vi "TubeTemperatures.vi"(9 "Startup Temperature (ºC)":dbl, 10 "TubeTempEnum":T1, 11 "Current Thermistor Temperatures":dbl[](array[numeric])) -> (3 "Current Tube Temperatures":dbl[](array[numeric]))   [LabVIEW 2019]
doc: "TubeTempNow = (temp of therm-TubeTempBefore) * t/RC)\nWhere t = 1s and RC = 128s\n\nRC was calculated emperically by James Sprenke for CPVC tubing.\nThe reason that RC is used is because it closely models the response from the temperature\nconduction from the sounding tube. This is not a theoretical derivation but a close \napproximation."
uses:
  TubeTempEnum.ctl
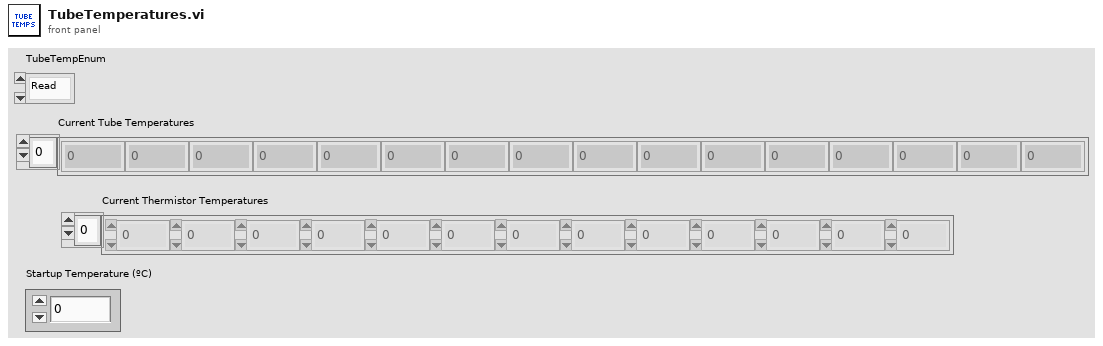
[diagram p1: front panel]
types:
  T1 = typedef "TubeTempEnum.ctl" = enum16{"Read", "Write", "Initialize"}
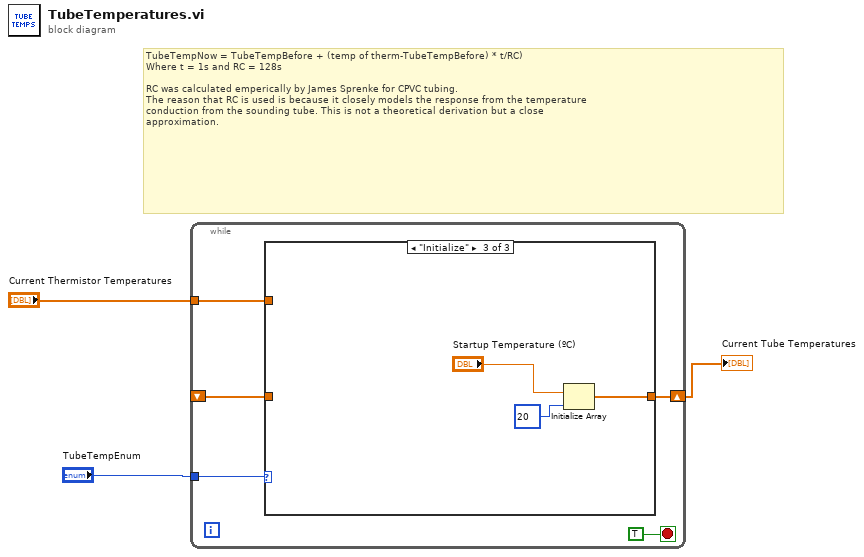
[diagram p0: block diagram]
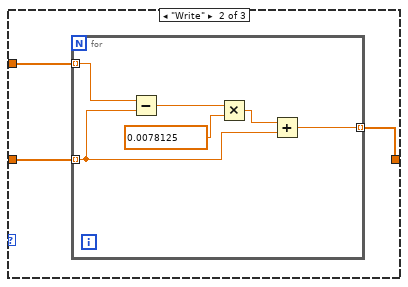
[diagram p3: hidden frame]
diagram:
  # "TubeTempNow = TubeTempBefore + (temp of therm-TubeTempBefore) * t/RC)\nWhere t = 1s and RC = 128s\n\nRC was calculated emperically by James Sprenke for CPVC tubing.\nThe reason that RC is used is because it closely models the response from the temperature\nconduction from the sounding tube. This is not a theoretical derivation but a close \napproximation."
  n1 = while {
    shift-right: [w5] -> w2
    shift-left: _ -> [w6]
    tunnel: "Current Thermistor Temperatures" -> [w7]
    tunnel: "TubeTempEnum" -> [w4]
    stop <- TRUE stop-if-true
    n2 = case shown="\"Initialize\"" w4 {
      tunnel: w7 -> [_ w12 _]
      tunnel: w6 -> [w9 w11 _]
      tunnel: [w9 w10 w19] -> w5
      frame "Read", Default {
      }
      frame "Write" {
        n3 = for {
          tunnel: w12 -> [w18] mode=indexing
          tunnel: w11 -> [w14] mode=indexing
          tunnel: [w15] -> w10 mode=indexing
          n4 = Subtract(x=w18, y=w14) -> (x-y=w17:dbl)
          n5 = Multiply(x=w17, y=0.0078125) -> (x*y=w13:dbl)
          n6 = Add(x=w13, y=w14) -> (x+y=w15:dbl)
        }
      }
      frame "Initialize" {
        n7 = Initialize Array("Startup Temperature (ºC)", 20 ("dimension size")) -> (w19:dbl[])
      }
    }
  }
  "Current Tube Temperatures" <- w2
